vi "发送Semantic_Dialogue_Array_Msg.vi"(7 "消息优先级（正常）":T2=enum."Normal", 8 "error in (no error)":cluster{"状态":bool, "代码":i32, "源":string} caption="错误输入（无错误）", 10 "值(信号)":T1, 11 "消息待入队列":refnum<class "Message Enqueuer.lvclass">) -> (0 "error out":cluster{"状态":bool, "代码":i32, "源":string} caption="错误输出", 3 "消息待入队列输出":refnum<class "Message Enqueuer.lvclass">)   [LabVIEW 2014, in "States.lvlib" / "Semantic_Dialogue_Array_Msg消息.lvclass"]
doc: "本VI将消息发送至操作者。"
uses:
  <vilib>/ActorFramework/Message Enqueuer/Message Enqueuer.lvclass
  <vilib>/ActorFramework/Message Enqueuer/Message Priority.ctl
  ctl/Semantic_Voice_Array.ctl
  <vilib>/ActorFramework/Message Enqueuer/Message Enqueuer.lvclass/Message Enqueuer.ctl
  <vilib>/ActorFramework/Message Priority Queue/Priority Enqueue.vi
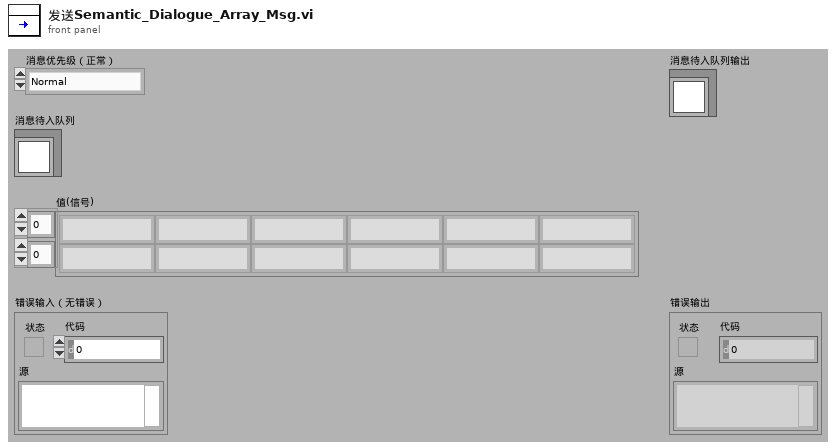
[diagram p1: front panel]
types:
  T1 = typedef "Semantic_Voice_Array.ctl" = string[][]
  T2 = typedef "Actor Framework.lvlib/Message Enqueuer.lvclass/Message Priority.ctl" = enum16{"Low", "Normal", "High"}
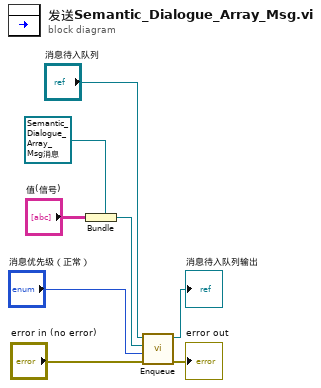
[diagram p0: block diagram]
diagram:
  n1 = Bundle(cluster=refnum<class "Semantic_Dialogue_Array_Msg消息.lvclass"> refnum ("Object"), "值(信号)") -> (w4:refnum<class "Semantic_Dialogue_Array_Msg消息.lvclass">)
  n2 = call <vilib>:"Enqueue.vi"("error in (no error)"="error in (no error)", "Message Priority (Normal)"="消息优先级（正常）", "Message"=w4, "Message Enqueuer in"="消息待入队列") -> ("error out"=→"error out":errorcluster, "Message Enqueuer out"=→"消息待入队列输出":refnum<class "Message Enqueuer.lvclass">)  [unwired: 6 in]
